vi "openWMPRef.vi"(8 "error in (no error)":errorcluster, 11 "SoundAO in":refnum<class "SoundAO.lvclass">) -> (0 "error out":errorcluster, 3 "SoundAO out":refnum<class "SoundAO.lvclass">)   [LabVIEW 2009, in "Hardware.lvlib" / "Channels.lvlib" / "SoundAO.lvclass"]
uses:
  SoundAO.lvclass
  SoundAO.lvclass/SoundAO.ctl
panel:
  in  "WindowsMediaPlayer":refnum<k7>(container)
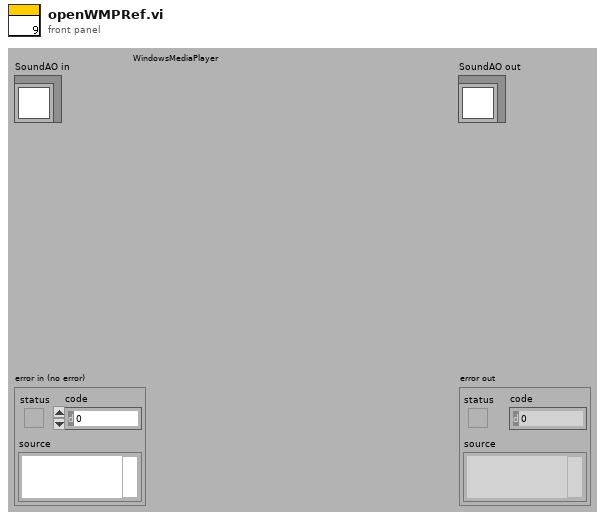
[diagram p1: front panel]
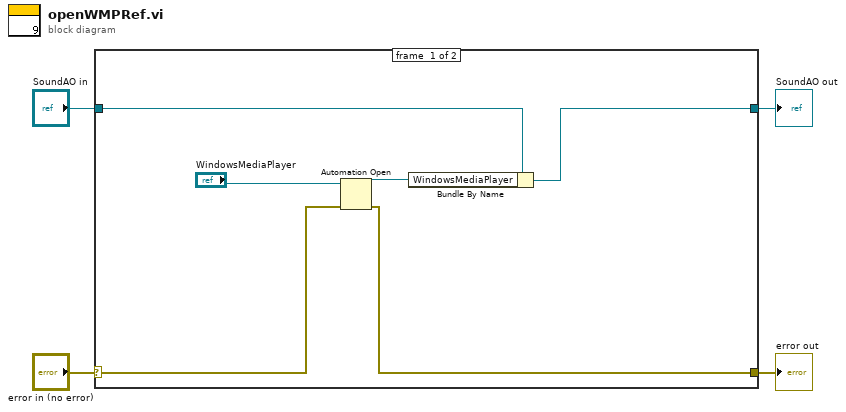
[diagram p0: block diagram]
diagram:
  n1 = case shown="No Error" "error in (no error)" {
    selector: "error in (no error)" -> [w10 w12]
    tunnel: [w6 w12] -> w3
    tunnel: [w7 w11] -> w1
    tunnel: "SoundAO in" -> [w8 w11]
    frame #0 {
      n2 = Automation Open(error in (no error)=w10, Automation Refnum="WindowsMediaPlayer") -> (Automation Refnum=w9:refnum<k7>, error out=w6:errorcluster)  [unwired: 2 in]
      n3 = Bundle By Name(cluster=w8, "WindowsMediaPlayer"=w9) -> (w7:refnum<class "SoundAO.lvclass">)
    }
    frame #1 {
    }
  }
  "error out" <- w3
  "SoundAO out" <- w1
